vi "replaceClusterElementByString.vi"(0 "cluster in":variant=variant(cluster{"DC Restore":enum16{"off", "on"}, "Polarity":enum16{"Negative", "Positive"}, "TV Event":enum16{"Field 1", "Field 2", "Any Field", "Any Line", "Line Number"}, "Coupling":enum16{"AC", "DC", "HF Reject", "LF Reject", "AC Plus HF Reject"}, "Slope":enum16{"Negative", "Positive"}, "Source":enum16{"Channel 0", "Channel 1", "External TRIG"}, "Window Mode":enum16{"Entering", "Leaving"}, "Low Level":dbl, "High Level":dbl, "Hysteresis":dbl, "Delay":dbl, "Holdoff":dbl, "Signal Format":enum16{"M-NTSC", "B/G-PAL", "SECAM", "M-PAL", "480i/59.94 fps", "480i/60 fps", "480p/59.94 Fps", "480p/60 Fps", "576i/50 fps", "576p/50 Fps", "720p/50 Fps", "720p/59.94 Fps", "720p/60 Fps", "1080i/50 fps", "1080i/59.94 fps", "1080i/60 fps", "1080p/24 Fps"}, "Mode":enum32{"Immediate", "Analog Edge", "Analog Window", "Analog Hysteresis", "Video", "Digital Edge"}, "Line Number":i32} {"DC Restore"=enum."off", "Polarity"=enum."Positive", "TV Event"=enum."Any Line", "Coupling"=enum."DC", "Slope"=enum."Positive", "Source"=enum."External TRIG", "Window Mode"=enum."Entering", "Low Level"=0.0, "High Level"=0.1, "Hysteresis"=0.05, "Delay"=0.0, "Holdoff"=0.0, "Signal Format"=enum."M-NTSC", "Mode"=enum."Immediate", "Line Number"=1}), 7 "Seperator (\"\")":string, 9 "Command":string="setTrigger.Mode", 11 "error in (no error)":errorcluster, 12 "setvalue":string="Analog Window") -> (4 "cluster out":variant=variant(cluster{"DC Restore":enum16{"off", "on"}, "Polarity":enum16{"Negative", "Positive"}, "TV Event":enum16{"Field 1", "Field 2", "Any Field", "Any Line", "Line Number"}, "Coupling":enum16{"AC", "DC", "HF Reject", "LF Reject", "AC Plus HF Reject"}, "Slope":enum16{"Negative", "Positive"}, "Source":enum16{"Channel 0", "Channel 1", "External TRIG"}, "Window Mode":enum16{"Entering", "Leaving"}, "Low Level":dbl, "High Level":dbl, "Hysteresis":dbl, "Delay":dbl, "Holdoff":dbl, "Signal Format":enum16{"M-NTSC", "B/G-PAL", "SECAM", "M-PAL", "480i/59.94 fps", "480i/60 fps", "480p/59.94 Fps", "480p/60 Fps", "576i/50 fps", "576p/50 Fps", "720p/50 Fps", "720p/59.94 Fps", "720p/60 Fps", "1080i/50 fps", "1080i/59.94 fps", "1080i/60 fps", "1080p/24 Fps"}, "Mode":enum32{"Immediate", "Analog Edge", "Analog Window", "Analog Hysteresis", "Video", "Digital Edge"}, "Line Number":i32} {"DC Restore"=enum."off", "Polarity"=enum."Positive", "TV Event"=enum."Any Line", "Coupling"=enum."DC", "Slope"=enum."Positive", "Source"=enum."External TRIG", "Window Mode"=enum."Entering", "Low Level"=0.0, "High Level"=0.1, "Hysteresis"=0.05, "Delay"=0.0, "Holdoff"=0.0, "Signal Format"=enum."M-NTSC", "Mode"=enum."Immediate", "Line Number"=1}), 8 "Seperator (\"\") out":string="Channel 1................................................", 15 "error out":errorcluster={"status"=TRUE, "code"=123, "source"="Error occurred during UpdateSettingAnCVT -  can not find \"Trigger.Mode\" in settingsCluster"})   [LabVIEW 2011]
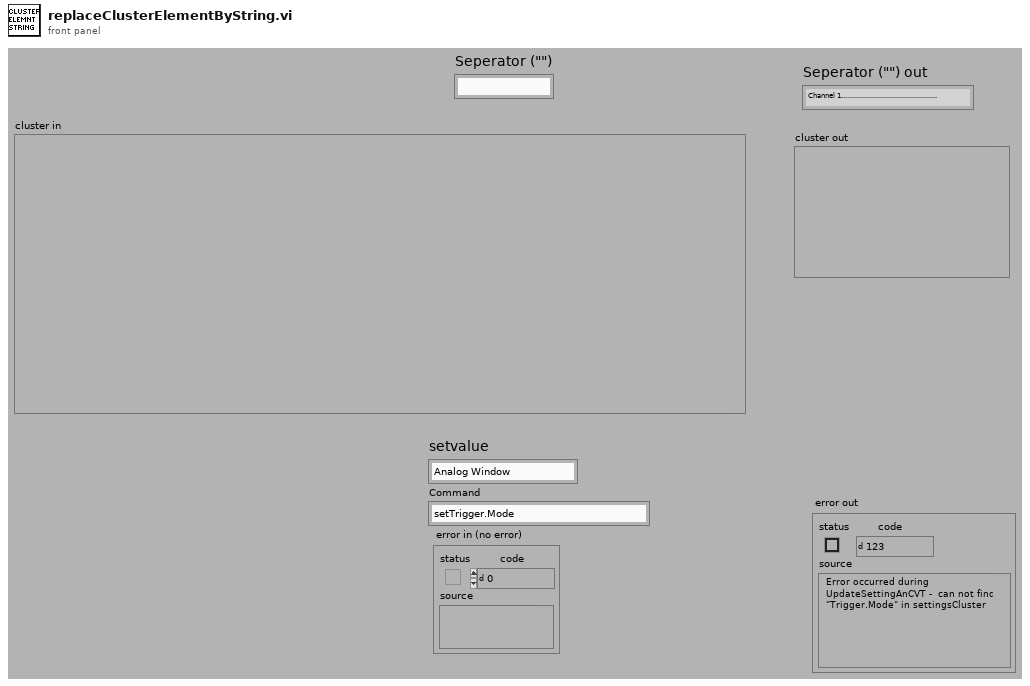
[diagram p1: front panel]
types:
  T1 = typedef "Type Descriptor Enumeration__ogtk.ctl" = enum8{"<Null>", "I8", "I16", "I32", "I64", "U8", "U16", "U32", "U64", "SGL", "DBL", "EXT", "CSG", "CDB", "CXT", "0x0F", "0x10", "0x11", "0x12", "0x13", "0x14", "Enum U8", "Enum U16", "Enum U32", "Enum U64", "SGL PQ", "DBL PQ", "EXT PQ", "CSG PQ", "CDB PQ", "CXT PQ", "0x1F", "0x20", "Boolean", "0x22", "0x23", "0x24", "0x25", "0x26", "0x27", "0x28", "0x29", "0x2A", "0x2B", "0x2C", "0x2D", "0x2E", "0x2F", "String", "0x31", "Path", "Pict", "0x34", "0x35", "0x36", "DAQ", "0x38", "0x39", "0x3A", "0x3B", "0x3C", "0x3D", "0x3E", "0x3F", "Array", "0x41", "0x42", "0x43", "0x44", "0x45", "0x46", "0x47", "0x48", "0x49", "0x4A", "0x4B", "0x4C", "0x4D", "0x4E", "0x4F", "Cluster", "0x51", "0x52", "Variant", "Waveform", "0x55", "0x56", "0x57", "0x58", "0x59", "0x5A", "0x5B", "0x5C", "0x5D", "0x5E", "0x5F", "0x60", "0x61", "0x62", "0x63", "0x64", "0x65", "0x66", "0x67", "0x68", "0x69", "0x6A", "0x6B", "0x6C", "0x6D", "0x6E", "0x6F", "Refnum"}
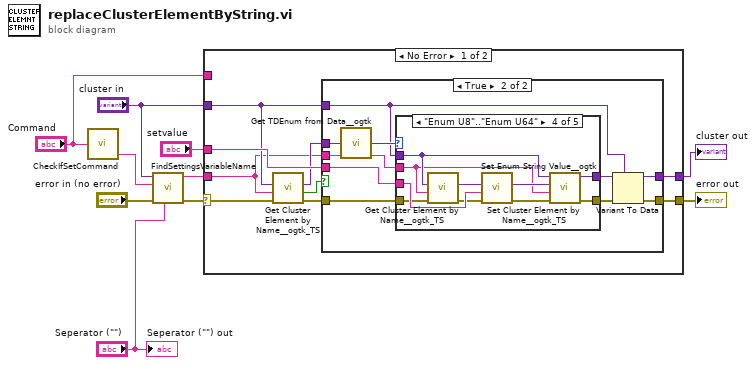
[diagram p0: block diagram]
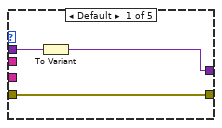
[diagram p3: hidden frame]
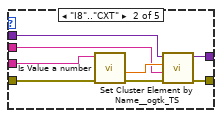
[diagram p4: hidden frame]
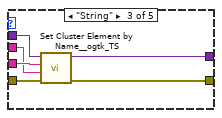
[diagram p5: hidden frame]
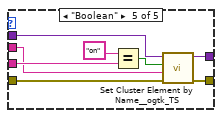
[diagram p6: hidden frame]
diagram:
  n1 = call "CheckIfSetCommand.vi"("Command"="Command") -> ("variable"=w6:string)  [unwired: 2 out]
  n2 = call "FindSettingsVariableName.vi"("Seperator (\"\")"="Seperator (\"\")", "error in (no error)"="error in (no error)", "variable"=w6, "variant"="cluster in") -> ("error out"=w5:errorcluster, "cluster name of variable"=w8:string)  [unwired: 6 in]
  n3 = case shown="No Error" w5 {
    selector: w5 -> [w15 w68]
    tunnel: "Command" -> [_ _]
    tunnel: "setvalue" -> [w19 _]
    tunnel: "cluster in" -> [w16 w67]
    tunnel: [w18 w68] -> w1
    tunnel: [w17 w67] -> w9
    tunnel: w8 -> [w11 _]
    frame No Error {
      n4 = call "Get Cluster Element by Name__ogtk_TS.vi"("error in (no error)"=w15, "Element Name"=w11, "Cluster"=w16) -> ("error out"=w14:errorcluster, "found?"=w12:bool, "VElement"=w13:variant)  [unwired: 6 in]
      n5 = case shown="True" w12 {
        tunnel: [w21 w31] -> w17
        tunnel: w19 -> [_ w30]
        tunnel: w16 -> [w21 w27]
        tunnel: w11 -> [_ w26]
        tunnel: w13 -> [_ w25]
        tunnel: w14 -> [w20 w24]
        tunnel: [w20 w22] -> w18
        frame False {
        }
        frame True {
          n6 = call "Get TDEnum from Data__ogtk.vi"("Data"=w25) -> ("Type Descriptor Enumeration"=w28:T1)  [unwired: 4 in]
          n7 = case shown="\"Enum U8\"..\"Enum U64\"" w28 {
            tunnel: w30 -> [_ w42 w47 w58 w66]
            tunnel: w27 -> [w34 w37 w48 w54 w65]
            tunnel: w26 -> [_ w39 w46 w52 w63]
            tunnel: [w33 w35 w43 w51 w62] -> w29
            tunnel: w24 -> [w32 w41 w45 w55 w64]
            tunnel: [w32 w36 w44 w50 w61] -> w23
            frame Default {
              n8 = To Variant(anything=w34) -> (Variant=w33:variant)
            }
            frame "I8".."CXT" {
              n9 = call "Is Value a number.vi"("user error in"=w41, "value String"=w42) -> ("user error out"=w38:errorcluster, "number"=w40:dbl)  [unwired: 6 in, 2 out]
              n10 = call "Set Cluster Element by Name__ogtk_TS.vi"("error in (no error)"=w38, "Element Name (\"\": New Element Data Name)"=w39, "New Element Value"=w40, "Cluster"=w37) -> ("error out"=w36:errorcluster, "VCluster out"=w35:variant)  [unwired: 5 in, 1 out]
            }
            frame "String" {
              n11 = call "Set Cluster Element by Name__ogtk_TS.vi"("error in (no error)"=w45, "Element Name (\"\": New Element Data Name)"=w46, "New Element Value"=w47, "Cluster"=w48) -> ("error out"=w44:errorcluster, "VCluster out"=w43:variant)  [unwired: 5 in, 1 out]
            }
            frame "Enum U8".."Enum U64" {
              n12 = call "Get Cluster Element by Name__ogtk_TS.vi"("error in (no error)"=w55, "Element Name"=w52, "Cluster"=w54) -> ("error out"=w56:errorcluster, "VElement"=w57:variant)  [unwired: 6 in, 1 out]
              n13 = call "Set Enum String Value__ogtk.vi"("error in (no error)"=w56, "String Value"=w58, "Default Enum Value"=w57) -> ("error out"=w49:errorcluster, "Enum"=w53:variant)  [unwired: 7 in]
              n14 = call "Set Cluster Element by Name__ogtk_TS.vi"("error in (no error)"=w49, "Element Name (\"\": New Element Data Name)"=w52, "New Element Value"=w53, "Cluster"=w54) -> ("error out"=w50:errorcluster, "VCluster out"=w51:variant)  [unwired: 5 in, 1 out]
            }
            frame "Boolean" {
              n15 = Equal?(x="on", y=w66) -> (x = y?=w59:bool)
              n16 = call "Set Cluster Element by Name__ogtk_TS.vi"("error in (no error)"=w64, "Element Name (\"\": New Element Data Name)"=w63, "New Element Value"=w59, "Cluster"=w65) -> ("error out"=w61:errorcluster, "VCluster out"=w62:variant)  [unwired: 5 in, 1 out]
            }
          }
          n17 = Variant To Data(error in=w23, type=w27, Variant=w29) -> (data=w31:variant, error out=w22:errorcluster)
        }
      }
    }
    frame Error {
    }
  }
  "error out" <- w1
  "cluster out" <- w9
  "Seperator (\"\") out" <- "Seperator (\"\")"
